vi "Induction Range Parse.vi"(8 "Error In":errorcluster, 11 "ERD Data Out":T1[](array[typedef])=[{"ERD Number"=62219, "Data"="01 F3 0B"}, {"ERD Number"=62246, "Data"="01 F3 26"}, {"ERD Number"=62247, "Data"="01 F3 27"}, {"ERD Number"=62723, "Data"="01 F5 03"}, {"ERD Number"=62724, "Data"="01 F5 04"}] {"ERD Number" format="%.0x"}) -> (0 "Error Out":errorcluster, 3 "Data":string[][](array[string]))   [LabVIEW 2016]
uses:
  Utility/LabVIEW GEA2 Toolkit v1.0.0.0/type defs/ERD Read Data Out.ctl
  Utility/LabVIEW GEA2 Toolkit v1.0.0.0/library/GEA2_Toolkit.lvlib
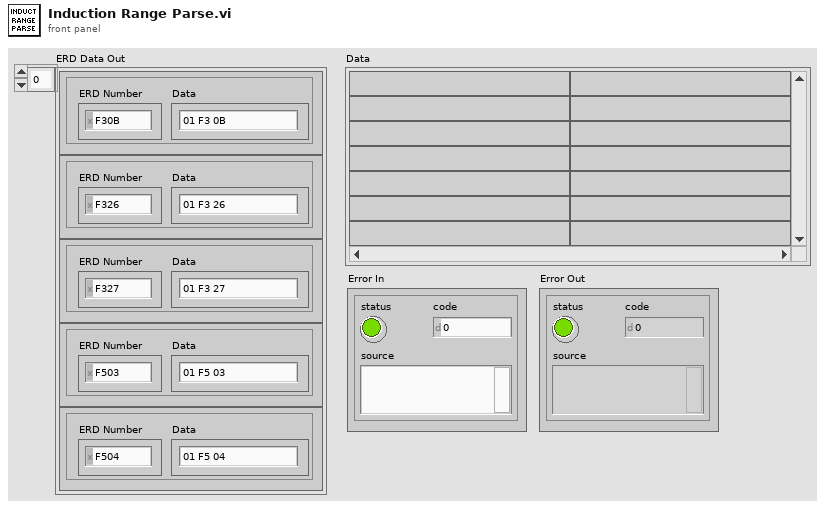
[diagram p1: front panel]
types:
  T1 = typedef "GEA2_Toolkit.lvlib/ERD Read Data Out.ctl" = cluster{"ERD Number":u16, "Data":string}
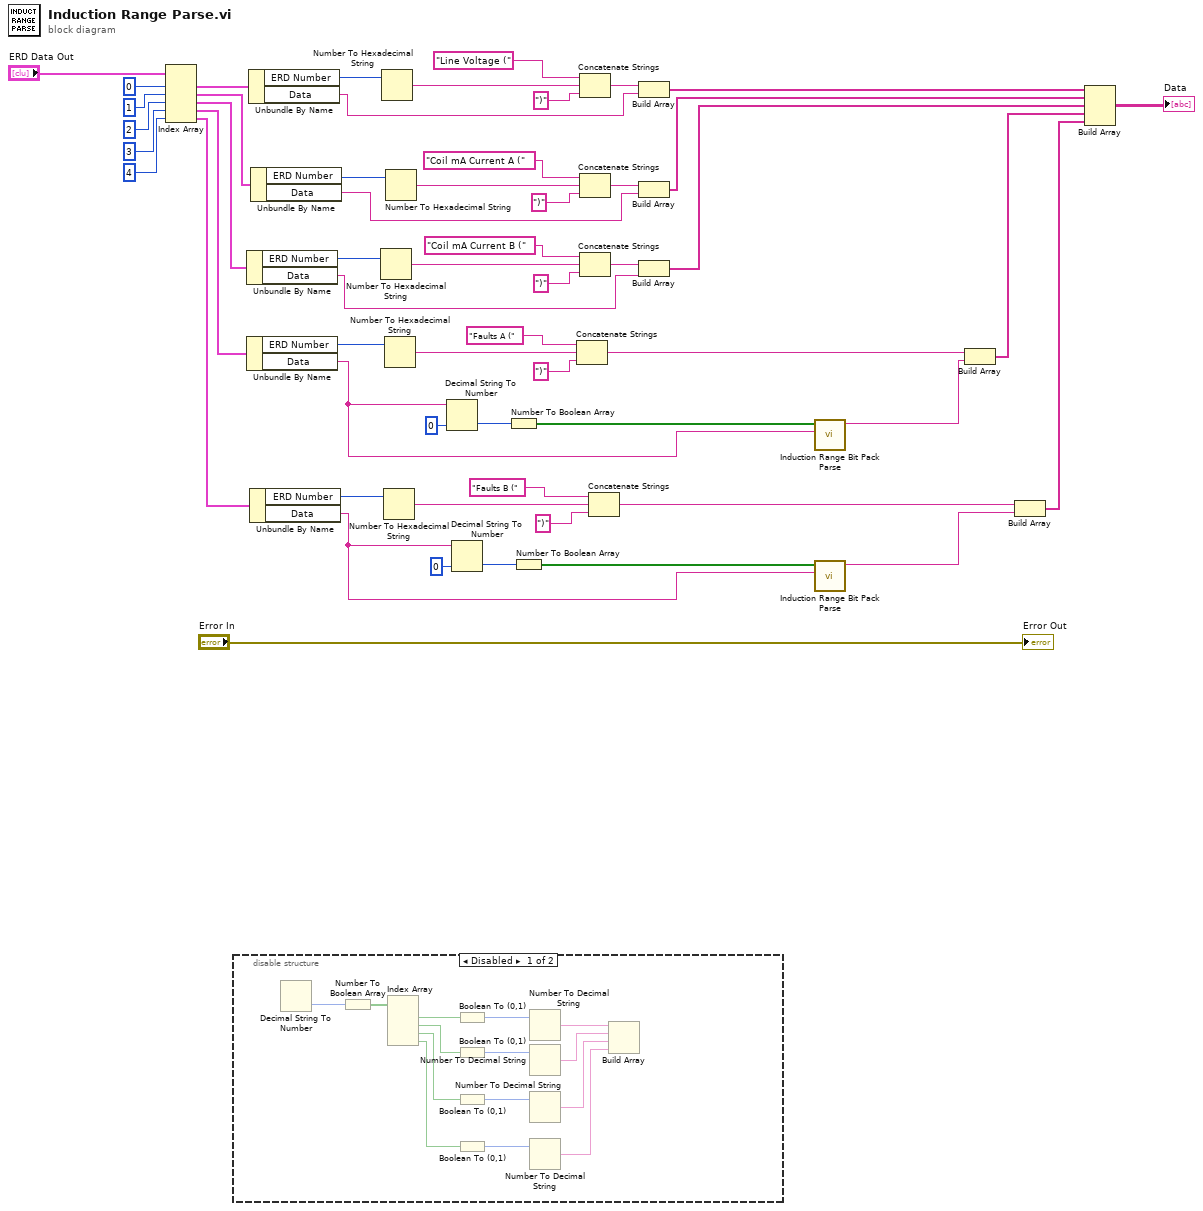
[diagram p0: block diagram]
diagram:
  n1 = Index Array(array="ERD Data Out", index #1=0 ("index"), index #2=1 ("index"), index #3=2 ("index"), index #4=3 ("index"), index #5=4 ("index")) -> (element #1=w26:T1, element #2=w15:T1, element #3=w14:T1, element #4=w13:T1, element #5=w12:T1)
  n2 = disable-structure shown="Disabled" {
    frame Disabled {
      n3 = Decimal String To Number() -> (number=w58:i32)  [unwired: 3 in, 1 out]
      n4 = Number To Boolean Array(number=w58) -> (Boolean array=w57:bool[])
      n5 = Index Array(array=w57) -> (element #1=w63:bool, element #2=w64:bool, element #3=w65:bool, element #4=w66:bool)  [unwired: 4 in]
      n6 = Boolean To (0,1)(Boolean=w63) -> (0, 1=w59:i16)
      n7 = Boolean To (0,1)(Boolean=w64) -> (0, 1=w60:i16)
      n8 = Boolean To (0,1)(Boolean=w65) -> (0, 1=w61:i16)
      n9 = Boolean To (0,1)(Boolean=w66) -> (0, 1=w62:i16)
      n10 = Number To Decimal String(number=w59) -> (decimal integer string=w67:string)  [unwired: 1 in]
      n11 = Number To Decimal String(number=w60) -> (decimal integer string=w68:string)  [unwired: 1 in]
      n12 = Number To Decimal String(number=w61) -> (decimal integer string=w69:string)  [unwired: 1 in]
      n13 = Number To Decimal String(number=w62) -> (decimal integer string=w70:string)  [unwired: 1 in]
      n14 = Build Array(w67, w68, w69, w70) -> ()  [unwired: 1 out]
    }
    frame Enabled {
    }
  }
  n15 = Unbundle By Name(w14) -> ("ERD Number"=w40:u16, "Data"=w17:string)
  n16 = Unbundle By Name(w13) -> ("ERD Number"=w44:u16, "Data"=w3:string)
  n17 = Unbundle By Name(w26) -> ("ERD Number"=w30:u16, "Data"=w5:string)
  n18 = Unbundle By Name(w12) -> ("ERD Number"=w50:u16, "Data"=w2:string)
  n19 = Unbundle By Name(w15) -> ("ERD Number"=w36:u16, "Data"=w18:string)
  n20 = Number To Hexadecimal String(2:w40) -> (0:w41:string)  [unwired: 1 in]
  n21 = Number To Hexadecimal String(2:w30) -> (0:w28:string)  [unwired: 1 in]
  n22 = Number To Hexadecimal String(2:w50) -> (0:w51:string)  [unwired: 1 in]
  n23 = Number To Hexadecimal String(2:w44) -> (0:w45:string)  [unwired: 1 in]
  n24 = Number To Hexadecimal String(2:w36) -> (0:w33:string)  [unwired: 1 in]
  n25 = Decimal String To Number(string=w3, default (0L)=u16 0 ("default (0 I32)")) -> (number=w11:u16)  [unwired: 1 in, 1 out]
  n26 = Decimal String To Number(string=w2, default (0L)=u16 0 ("default (0 I32)")) -> (number=w6:u16)  [unwired: 1 in, 1 out]
  n27 = Number To Boolean Array(number=w11) -> (Boolean array=w9:bool[])
  n28 = Number To Boolean Array(number=w6) -> (Boolean array=w4:bool[])
  n29 = Concatenate Strings("Faults A (", w45, ")" ("string")) -> (w43:string)
  n30 = Concatenate Strings("Line Voltage (", w28, ")" ("string")) -> (w31:string)
  n31 = Concatenate Strings("Coil mA Current A (", w33, ")" ("string")) -> (w35:string)
  n32 = Concatenate Strings("Coil mA Current B (", w41, ")" ("string")) -> (w37:string)
  n33 = Concatenate Strings("Faults B (", w51, ")" ("string")) -> (w48:string)
  n34 = Build Array(w31, w5) -> (w52:string[])
  n35 = Build Array(w35, w18) -> (w53:string[])
  n36 = Build Array(w37, w17) -> (w54:string[])
  n37 = call "Induction Range Bit Pack Parse.vi"("Raw Data"=w3, "Boolean array"=w9) -> ("String"=w8:string)  [unwired: 9 in]
  n38 = call "Induction Range Bit Pack Parse.vi"("Raw Data"=w2, "Boolean array"=w4) -> ("String"=w1:string)  [unwired: 9 in]
  n39 = Build Array(w43, w8) -> (w55:string[])
  n40 = Build Array(w48, w1) -> (w56:string[])
  n41 = Build Array(w52, w53, w54, w55, w56) -> (→"Data":string[][])
  "Error Out" <- "Error In"
